vi "Connector.vi"(8 "error in":errorcluster, 10 "Sporks number":i32, 11 "VISA resource name":refnum<visa-resource-name>) -> (0 "error out":errorcluster, 1 "Measurement":i32[](array[numeric]), 2 "Spoke":i32[](array[numeric]), 3 "First spoke side":T1, 5 "Instrument IDN":string)   [LabVIEW 2025]
uses:
  Controls/Spoke_side.ctl
panel:
  out "No response":bool
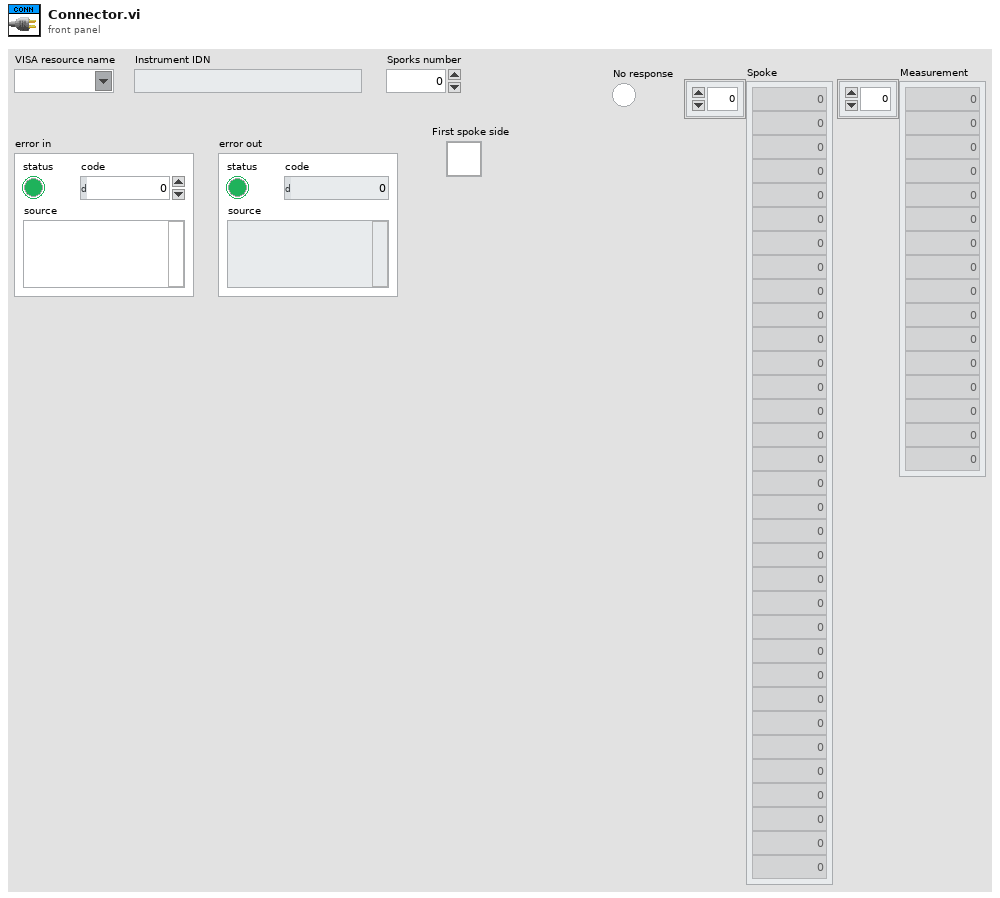
[diagram p1: front panel]
types:
  T1 = typedef "Spoke_side.ctl" = u16
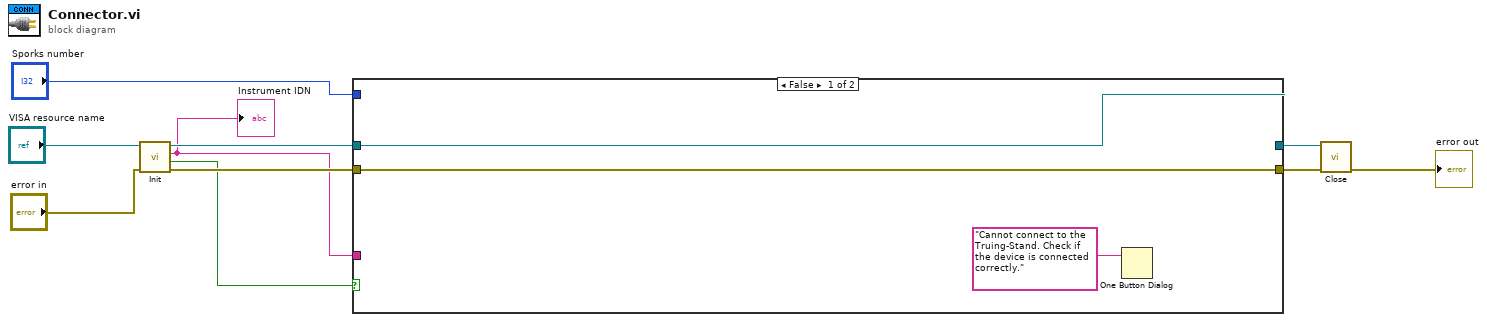
[diagram p0: block diagram]
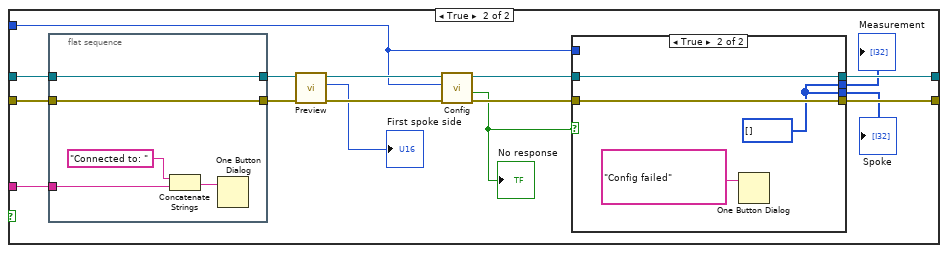
[diagram p2: hidden frame]
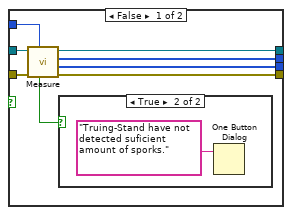
[diagram p3: hidden frame]
diagram:
  n1 = call "Init.vi"("error in"="error in", "VISA resource in"="VISA resource name") -> ("error out"=w8:errorcluster, "Passed Init?"=w7:bool, "Instrument IDN"=w1:string, "VISA resource out"=w10:refnum<visa-resource-name>)  [unwired: 6 in]
  "Instrument IDN" <- w1
  n2 = case shown="False" w7 {
    tunnel: w10 -> [w13 w16]
    tunnel: [w12 w29] -> w5
    tunnel: [w13 w28] -> w6
    tunnel: w8 -> [w12 w18]
    tunnel: "Sporks number" -> [_ w19]
    tunnel: w1 -> [_ w20]
    frame False {
      n3 = One Button Dialog(message="Cannot connect to the Truing-Stand. Check if the device is connected correctly.") -> ()  [unwired: 1 in, 1 out]
    }
    frame True {
      n4 = flat-sequence {
        tunnel: w20 -> [w34]
        tunnel: w18 -> [w31]
        tunnel: [w31] -> w17
        tunnel: w16 -> [w30]
        tunnel: [w30] -> w15
        frame #0 {
          n5 = Concatenate Strings("Connected to: " ("string"), w34) -> (w32:string)
          n6 = One Button Dialog(message=w32) -> ()  [unwired: 1 in, 1 out]
        }
      }
      n7 = call "Preview.vi"("error in"=w17, "VISA resource in"=w15) -> ("error out"=w23:errorcluster, "First spoke side"=→"First spoke side":T1, "VISA resource out"=w22:refnum<visa-resource-name>)  [unwired: 7 in]
      n8 = call "Config.vi"("error in"=w23, "Sporks Number"=w19, "VISA resource in"=w22) -> ("error out"=w25:errorcluster, "No response"=w21:bool, "VISA resource out"=w24:refnum<visa-resource-name>)  [unwired: 6 in]
      "No response" <- w21
      n9 = case shown="True" w21 {
        tunnel: [w42 w47] -> w29
        tunnel: [w41 w46] -> w28
        tunnel: [w40 w45] -> w27
        tunnel: [w39 w45] -> w26
        tunnel: w25 -> [w37 w47]
        tunnel: w24 -> [w36 w46]
        tunnel: w19 -> [w35 _]
        frame False {
          n10 = call "Measure.vi"("Sporks Number"=w35, "error in"=w37, "VISA resource in"=w36) -> ("error out"=w42:errorcluster, "Spork"=w39:i32[], "Deviation"=w40:i32[], "VISA resource out"=w41:refnum<visa-resource-name>, "Timeout"=w38:bool)  [unwired: 4 in]
          n11 = case shown="True" w38 {
            frame False {
            }
            frame True {
              n12 = One Button Dialog(message="Truing-Stand have not detected suficient amount of sporks.") -> ()  [unwired: 1 in, 1 out]
            }
          }
        }
        frame True {
          w45 = i32[] [] ("Deviation")
          n13 = One Button Dialog(message="Config failed") -> ()  [unwired: 1 in, 1 out]
        }
      }
      "Measurement" <- w27
      "Spoke" <- w26
    }
  }
  n14 = call "Close.vi"("error in"=w5, "VISA resource in"=w6) -> ("error out"=→"error out":errorcluster)  [unwired: 9 in]
